vi "Get gRPC ID.vi"(11 "OOP Server in":refnum<class "Servicer.lvclass">) -> (2 "gRPC ID":T1, 3 "OOP Server out":refnum<class "Servicer.lvclass">)   [LabVIEW 2019, in "gRPC-servicer.lvlib" / "Servicer.lvclass"]
uses:
  Servicer.lvclass
  LabVIEW gRPC Library/Shared/grpcId.ctl
  Servicer.lvclass/Servicer.ctl
  LabVIEW gRPC Library/grpc-lvsupport.lvlib
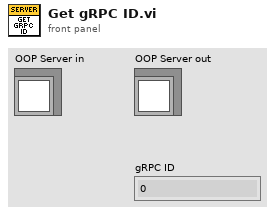
[diagram p1: front panel]
types:
  T1 = typedef "grpc-lvsupport.lvlib/grpcId.ctl" = u64
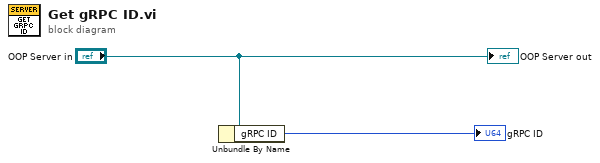
[diagram p0: block diagram]
diagram:
  n1 = Unbundle By Name("OOP Server in") -> ("gRPC ID"=→"gRPC ID":T1)
  "OOP Server out" <- "OOP Server in"
